vi "getPoints.vi"(0 "reference":refnum<class "SegmentedLineEdge.lvclass">, 5 "error in (no error)":errorcluster) -> (14 "reference out":refnum<class "SegmentedLineEdge.lvclass">, 15 "points":T1[](array[typedef]) {"y" format="%.2f"; "x" format="%.2f"}, 19 "error out":errorcluster)   [LabVIEW 2014, in "SegmentedLineEdge.lvclass"]
doc: "Abstract getPoints"
uses:
  <resource>/Framework/Providers/Open_GDS/UML/SegmentedLineEdge_class/SegmentedLineEdge.lvclass
  <resource>/Framework/Providers/Open_GDS/UML/General/Point/Point Point2D.ctl
  <resource>/Framework/Providers/Open_GDS/UML/AbstractNode_class/AbstractNode.lvclass
  <resource>/Framework/Providers/Open_GDS/UML/Direction_class/Direction.lvclass
  <resource>/Framework/Providers/Open_GDS/UML/AbstractEdge_class/AbstractEdge.lvclass
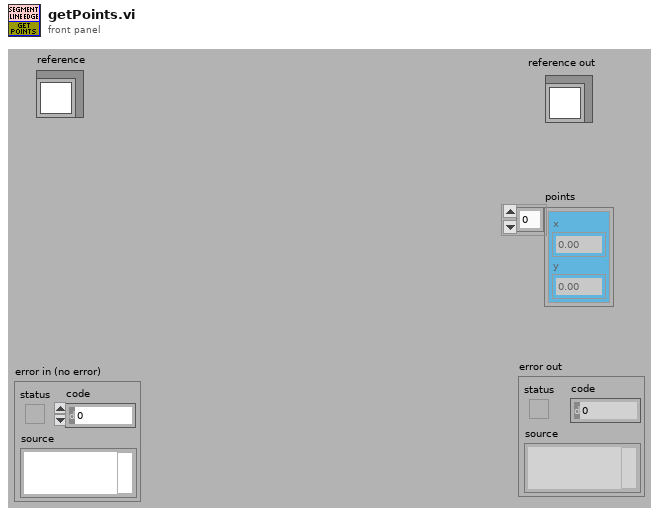
[diagram p1: front panel]
types:
  T1 = typedef "Point Point2D.ctl" = cluster{"x":dbl, "y":dbl}
  T2 = typedef "AbstractEdge.lvclass/ObjectAttributes.ctl" = cluster{"start":refnum<class "AbstractNode.lvclass">, "end":refnum<class "AbstractNode.lvclass">}
  T3 = typedef "Rectangle Rectangle2D.ctl" = cluster{"x":dbl, "y":dbl, "width":dbl, "height":dbl}
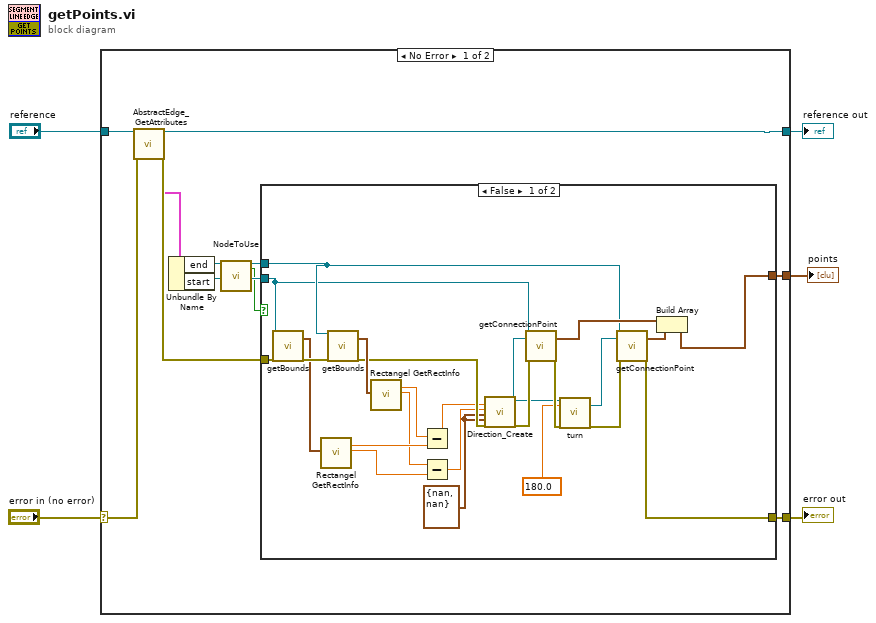
[diagram p0: block diagram]
diagram:
  n1 = case shown="No Error" "error in (no error)" {
    selector: "error in (no error)" -> [w14 w43]
    tunnel: "reference" -> [w17 w44]
    tunnel: [w16 w43] -> w4
    tunnel: [w15 w44] -> w3
    tunnel: [w13 _] -> w1
    frame No Error {
      n2 = call <resource>:"AbstractEdge_GetAttributes.vi"("reference in"=w17, "error in (no error)"=w14) -> ("reference out"=w15:refnum<class "SegmentedLineEdge.lvclass">, "Data"=w6:T2, "error out"=w12:errorcluster)  [unwired: 14 in, 1 out]
      n3 = Unbundle By Name(w6) -> ("end"=w11:refnum<class "AbstractNode.lvclass">, "start"=w9:refnum<class "AbstractNode.lvclass">)
      n4 = call <resource>:"NodeToUse.vi"("reference in"=w11, "reference in 2"=w9) -> ("reference out"=w10:refnum<class "AbstractNode.lvclass">, "Same"=w7:bool, "reference out 2"=w8:refnum<class "AbstractNode.lvclass">)  [unwired: 14 in, 1 out]
      n5 = case shown="False" w7 {
        tunnel: [w18 w42] -> w16
        tunnel: [w41 _] -> w13
        tunnel: w12 -> [w22 w42]
        tunnel: w10 -> [w21 _]
        tunnel: w8 -> [w20 _]
        frame False {
          w19 = T1 {"x"=nan, "y"=nan} ("p1")
          n6 = call-dynamic "getBounds.vi"("reference"=w20, "error in (no error)"=w22) -> ("bounds"=w39:T3, "error out"=w40:errorcluster)  [unwired: 15 in, 1 out]
          n7 = call <resource>:"Rectangel GetRectInfo.vi"("bounds"=w39) -> ("centerX"=w27:dbl, "centerY"=w25:dbl)  [unwired: 1 in, 16 out]
          n8 = call-dynamic "getBounds.vi"("reference"=w21, "error in (no error)"=w40) -> ("bounds"=w38:T3, "error out"=w37:errorcluster)  [unwired: 15 in, 1 out]
          n9 = call <resource>:"Rectangel GetRectInfo.vi"("bounds"=w38) -> ("centerX"=w28:dbl, "centerY"=w26:dbl)  [unwired: 1 in, 16 out]
          n10 = Subtract(x=w28, y=w27) -> (x-y=w24:dbl)
          n11 = Subtract(x=w26, y=w25) -> (x-y=w23:dbl)
          n12 = call <resource>:"Direction_Create.vi"("dx"=w24, "dy"=w23, "p1"=w19, "p2"=w19, "error in (no error)"=w37) -> ("reference out"=w31:refnum<class "Direction.lvclass">, "error out"=w34:errorcluster)  [unwired: 13 in]
          n13 = call-dynamic "getConnectionPoint.vi"("reference"=w20, "direction"=w31, "error in (no error)"=w34) -> ("point2D"=w36:T1, "error out"=w32:errorcluster)  [unwired: 14 in, 1 out]
          n14 = call <resource>:"turn.vi"("reference"=w31, "angle"=180.0 ("degrees"), "error in (no error)"=w32) -> ("turnedDirection"=w29:refnum<class "Direction.lvclass">, "error out"=w33:errorcluster)  [unwired: 15 out]
          n15 = call-dynamic "getConnectionPoint.vi"("reference"=w21, "direction"=w29, "error in (no error)"=w33) -> ("point2D"=w35:T1, "error out"=w18:errorcluster)  [unwired: 14 in, 1 out]
          n16 = Build Array(w36, w35) -> (w41:T1[])
        }
        frame True {
        }
      }
    }
    frame Error {
    }
  }
  "reference out" <- w3
  "error out" <- w4
  "points" <- w1
